vi "Read Is Client.vi"(8 "error in (no error)":errorcluster, 11 "WebSocket Client in":refnum<class "WebSocket Client.lvclass">) -> (0 "error out":errorcluster, 2 "Is Client":bool, 3 "WebSocket Client out":refnum<class "WebSocket Client.lvclass">)   [LabVIEW 2021, in "WebSocket Actors.lvlib" / "WebSocket Client.lvclass"]
uses:
  WebSocket Client.lvclass
  WebSocket Client.lvclass/WebSocket Client.ctl
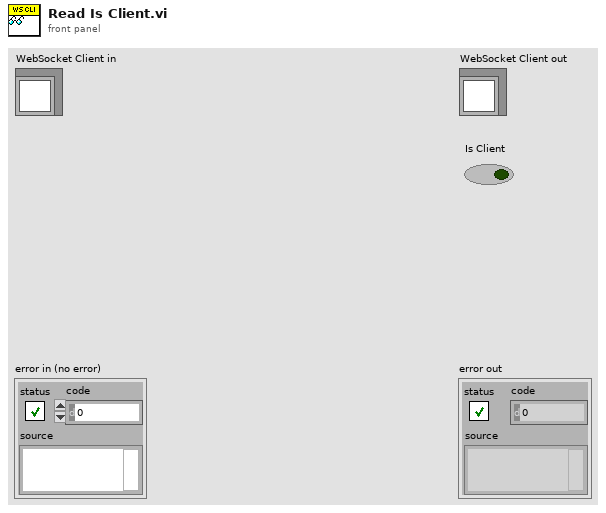
[diagram p1: front panel]
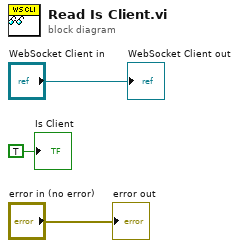
[diagram p0: block diagram]
diagram:
  "error out" <- "error in (no error)"
  "WebSocket Client out" <- "WebSocket Client in"
  "Is Client" <- TRUE ("Is Client")
